vi "ActiveObjects_QueueQueue_SendMsgToProcess_4x4x4_Singleton.vi"(8 "Error In":errorcluster, 10 "MessageToProcess":string) -> (0 "Error Out":errorcluster)   [LabVIEW 2020]
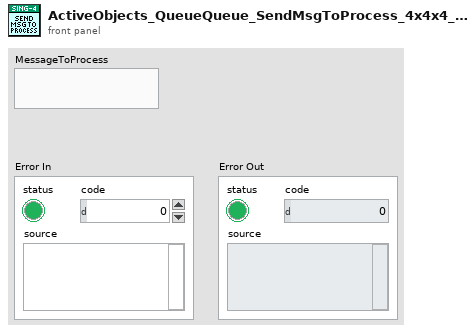
[diagram p1: front panel]
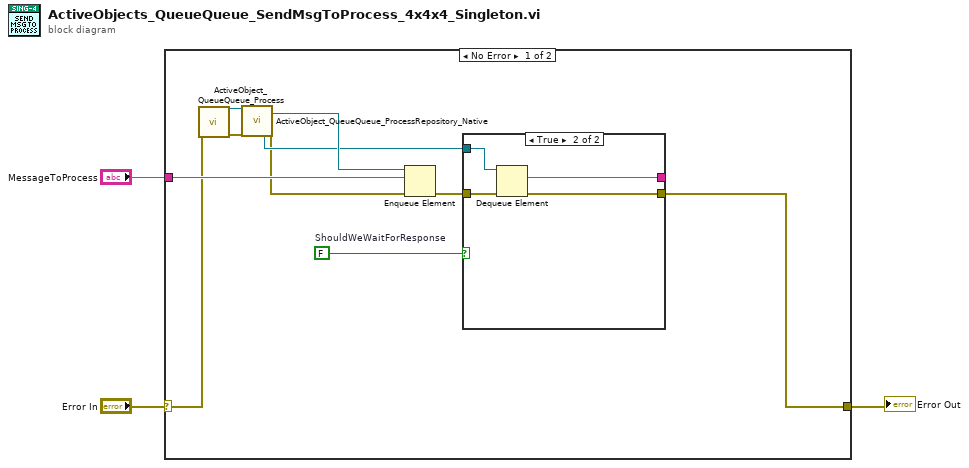
[diagram p0: block diagram]
diagram:
  n1 = case shown="No Error" "Error In" {
    selector: "Error In" -> [w5 w19]
    tunnel: [w7 w19] -> w2
    tunnel: "MessageToProcess" -> [w12 _]
    frame No Error {
      w11 = FALSE  # ShouldWeWaitForResponse
      n2 = call "ActiveObject_QueueQueue_Process.vi"("Error In"=w5) -> ("reference out"=w6:refnum<class>, "Error Out"=w4:errorcluster)  [unwired: 17 in]
      n3 = call "ActiveObject_QueueQueue_ProcessRepository_Native.vi"("reference in"=w6, "Error In"=w4) -> ("FromProcessQueue"=w9:refnum<queue>, "ToProcessQueue"=w13:refnum<queue>, "Error Out"=w8:errorcluster)  [unwired: 11 in, 4 out]
      n4 = Enqueue Element(queue=w13, element=w12, error in (no error)=w8) -> (error out=w10:errorcluster)  [unwired: 1 in, 2 out]
      n5 = case shown="True" w11 {
        tunnel: w10 -> [w14 w18]
        tunnel: w9 -> [_ w17]
        tunnel: [_ w16] -> _
        tunnel: [w14 w15] -> w7
        frame False {
        }
        frame True {
          n6 = Dequeue Element(queue=w17, error in (no error)=w18) -> (element=w16:string, error out=w15:errorcluster)  [unwired: 1 in, 2 out]
        }
      }
    }
    frame Error {
    }
  }
  "Error Out" <- w2
